vi "Configure Filter.vi"   [LabVIEW 2021, in "Yokogawa WT1800 Series.lvlib"]
doc: "Configures the filter features."
uses:
  <instrlib>/Yokogawa WT1800 Series/Yokogawa WT1800 Series.lvlib
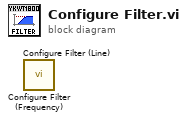
[diagram p0: block diagram]
diagram:
  n1 = call <instrlib>:"Configure Filter (Frequency).vi"() -> ()  [unwired: 10 in, 2 out]
  n2 = call <instrlib>:"Configure Filter (Line).vi"() -> ()  [unwired: 10 in, 2 out]
